vi "Field Draw Paths.vi"(4 "Draw Targets?":T2, 6 "Lado":enum16{"Esquerdo", "Direito"}(ring), 7 "RobotRef":refnum<class "Robot.lvclass">[](array[class]), 8 "Offset":T1, 9 "Scale mm/pixel":dbl, 11 "picture in":picture) -> (3 "picture out":picture)   [LabVIEW 2022 SP3]
uses:
  Robot_class/Robot.lvclass
  DrawTargets.ctl
  <vilib>/Utility/miscctls.llb/LVBoundsTypeDef.ctl
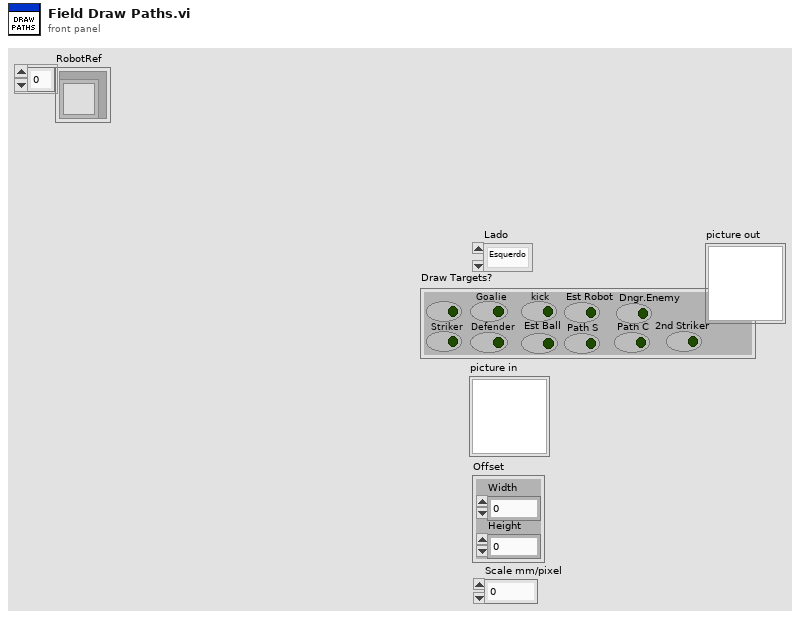
[diagram p1: front panel]
types:
  T1 = typedef "LVBoundsTypeDef.ctl" = cluster{"Width":u32, "Height":u32}
  T2 = typedef "DrawTargets.ctl" = cluster{"Attacker":bool, "Striker":bool, "Goalie":bool, "Defender":bool, "kick":bool, "Est Ball":bool, "Est Robot":bool, "Path S":bool, "Path C":bool, "Dngr.Enemy":bool, "2nd Striker":bool}
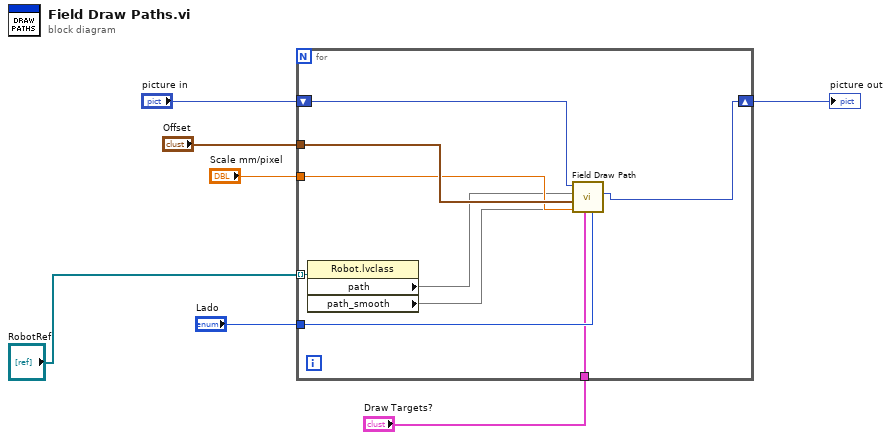
[diagram p0: block diagram]
diagram:
  n1 = for {
    tunnel: "Lado" -> [w16]
    tunnel: "Draw Targets?" -> [w15]
    tunnel: "Offset" -> [w13]
    tunnel: "Scale mm/pixel" -> [w12]
    shift-right: [w11] -> w2
    shift-left: "picture in" -> [w14]
    tunnel: "RobotRef" -> [w10] mode=indexing
    n2 = property class="Robot.lvclass"(reference=w10) -> ("path"=w9, "path_smooth"=w8)  [unwired: 1 in, 2 out]
    n3 = call "Field Draw Path.vi"("Pontos Smooth"=w8, "Lado"=w16, "Draw Targets?"=w15, "Scale mm/pixel"=w12, "Offset"=w13, "Pontos"=w9, "picture in"=w14) -> ("picture out"=w11:picture)  [unwired: 4 in]
  }
  "picture out" <- w2
